vi "GageComplexTriggerAcquire.vi"() -> ()   [LabVIEW 2015]
panel:
  in  "Force":bool
  in  "Trigger Engines":T1(array[cluster])=[{"Slope"=0, "Level"=0, "Source"=0, "External Range"=2000, "External Coupling"=0, "External"=FALSE, "Disable"=FALSE, "External Impedance"=1}] {"External Impedance" items=["50 Ohm", "HiZ"]; "External Coupling" items=["DC", "AC"]; "External Range" min=2000 max=10000 step=8000; "Slope" items=["Rising", "Falling"]; "Level" min=-100 max=100; "Source" min=0 max=64 step=1}
  in  "Channels":T2(array[cluster])=[{"Coupling"=0, "Differential Input"=FALSE, "Direct-to-ADC"=FALSE, "Range"=2000, "Impedance"=50, "DC Offset"=0, "Filter"=0}] {"Impedance" min=50 max=1000000 step=999950; "Coupling" items=["DC", "AC"]}
  in  "Acquisition":T3={"Sample Rate"=100000000.0, "Mode"=0, "Depth"=8192.0, "Segment Size"=8192.0, "Trigger Timeout"=1000000.0, "Trigger Holdoff"=0.0, "Trigger Delay"=0.0, "Clock mode"=enum."Internal"} {"Segment Size" min=256.0 step=128.0; "Trigger Delay" min=0.0 step=128.0; "Trigger Holdoff" min=0.0 step=128.0; "Depth" min=256.0 step=128.0; "Mode" items=["Single", "Dual", "Quad", "Octal"]}
  in  "Continuous":bool
  out "Progress":string
  in  "stop":bool
  out "Waveform Graph":cluster{dbl, dbl, "Data in Volts":dbl[][]}(graph)
  out "System Name":string
  out "Sample Bits":i32
  out "Trigger Count":i32
  out "Channel Count":i32
  out "Board Count":i32
  out "System Count":i32
  in  "Points":u32=4096
  in  "Start":i32
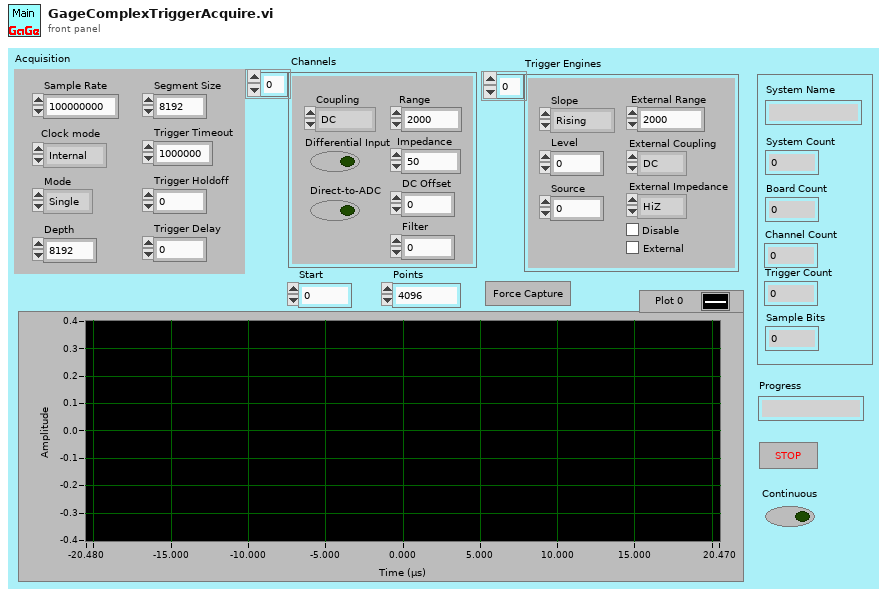
[diagram p1: front panel]
types:
  T1 = cluster{"Slope":u16, "Level":i32, "Source":i32, "External Range":u32, "External Coupling":u16, "External":bool, "Disable":bool, "External Impedance":u16}[]
  T2 = cluster{"Coupling":u16, "Differential Input":bool, "Direct-to-ADC":bool, "Range":u32, "Impedance":u32, "DC Offset":i32, "Filter":i32}[]
  T3 = cluster{"Sample Rate":dbl, "Mode":u16, "Depth":dbl, "Segment Size":dbl, "Trigger Timeout":dbl, "Trigger Holdoff":dbl, "Trigger Delay":dbl, "Clock mode":enum16{"Internal", "External", "Reference"}}
  T4 = cluster{"Handle":u32, "Sample size":u32, "Resolution":i32, "Offset":i32, "Channels":u32, "Boards":u32}
  T5 = cluster{"Slope":u16, "Level":i32, "Source":i32, "External Range":u32, "External Coupling":u16, "External":bool, "Disable":bool, "External Impedance":u16}
  T6 = cluster{"Coupling":u16, "Differential Input":bool, "Direct-to-ADC":bool, "Range":u32, "Impedance":u32, "DC Offset":i32, "Filter":i32}
  T7 = cluster{string, "Level":i32, "Source":i32, "External Range":u32, string, "External":bool, "Disable":bool, string}
  T8 = cluster{string, "Differential Input":bool, "Direct-to-ADC":bool, "Range":u32, "Impedance":u32, "DC Offset":i32, "Coupling":u16}
  T9 = cluster{"Sample Rate":dbl, "Clock mode":enum16{"Internal", "External", "Reference"}, "RingText.Text":string, "Depth":dbl, "Segment Size":dbl, "Trigger Timeout":dbl, "Trigger Holdoff":dbl, "Trigger Delay":dbl}
  T10 = cluster{"Handle":u32, "Sample Size":u32, "Resolution":i32, "Offset":i32, "Channels":u32, "Boards":u32}
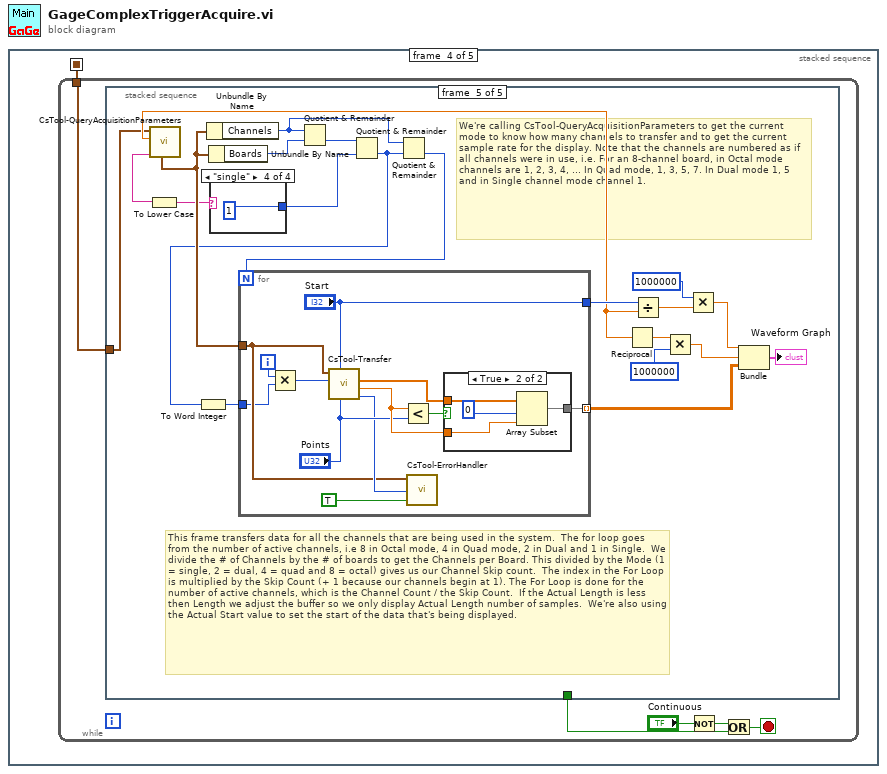
[diagram p0: block diagram]
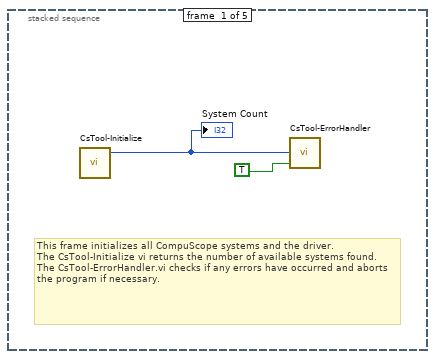
[diagram p2: hidden frame]
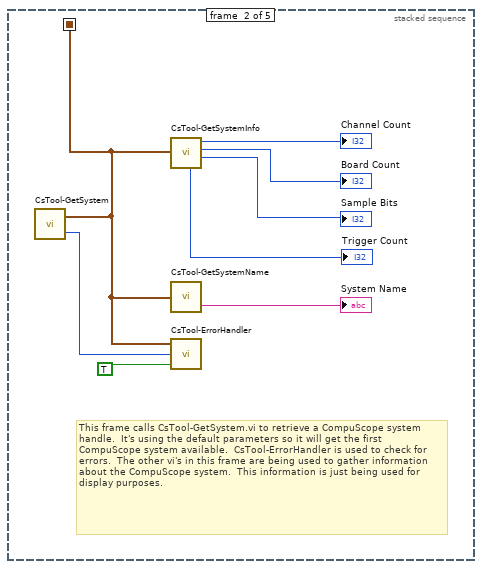
[diagram p3: hidden frame]
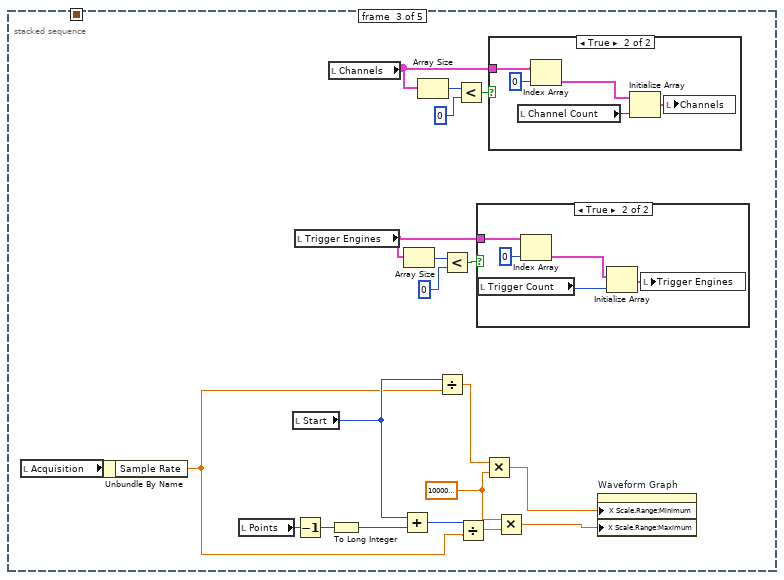
[diagram p4: hidden frame]
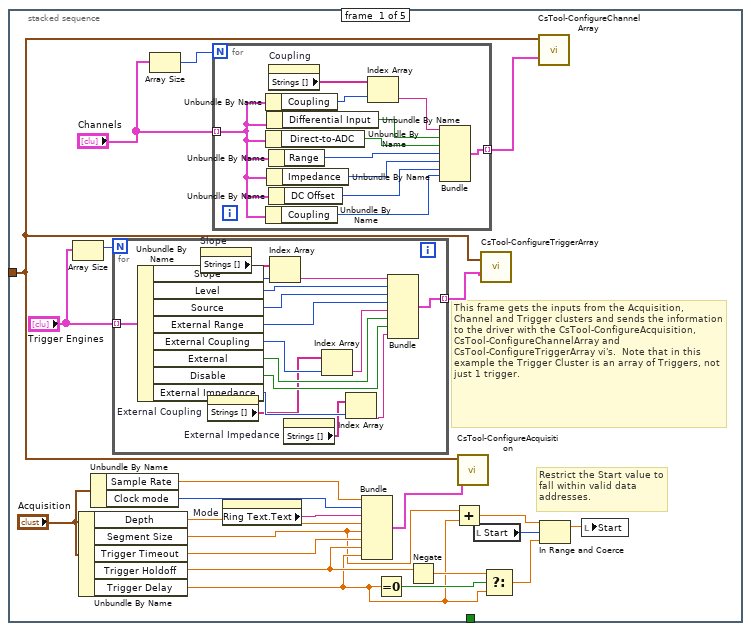
[diagram p7: hidden frame]
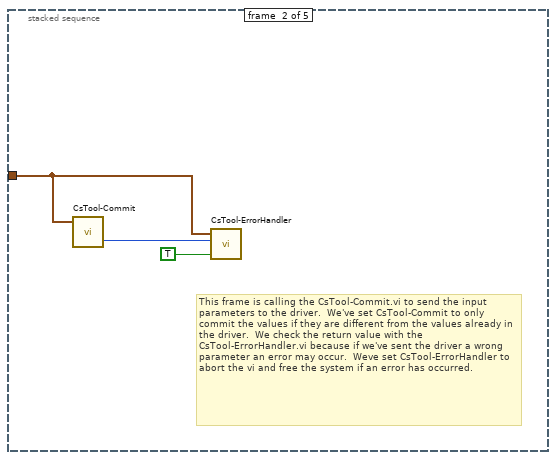
[diagram p8: hidden frame]
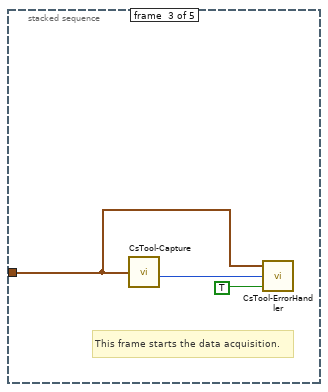
[diagram p9: hidden frame]
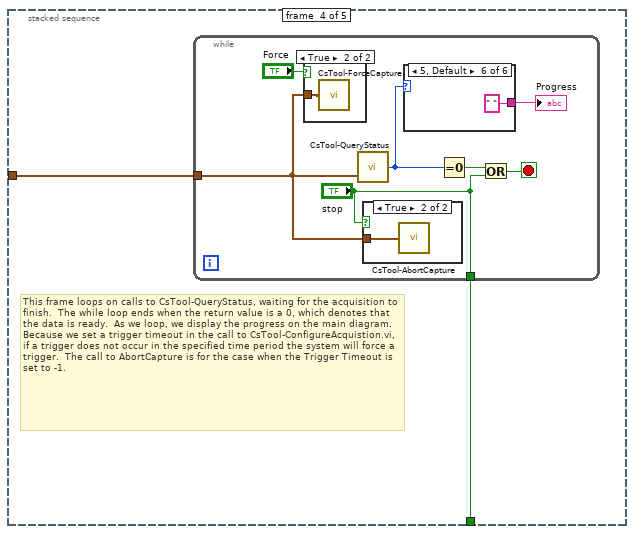
[diagram p10: hidden frame]
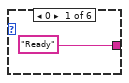
[diagram p13: hidden frame]
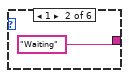
[diagram p14: hidden frame]
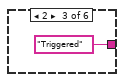
[diagram p15: hidden frame]
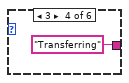
[diagram p16: hidden frame]
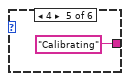
[diagram p17: hidden frame]
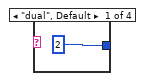
[diagram p18: hidden frame]
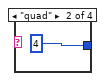
[diagram p19: hidden frame]
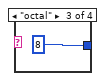
[diagram p20: hidden frame]
diagram:
  n1 = stacked-sequence {
    seq-local: [_ w5 _ _ _] -> [_ _ _ w41 w162]
    frame #0 {
      # "This frame initializes all CompuScope systems and the driver.\nThe CsTool-Initialize vi returns the number of available systems found.  The CsTool-ErrorHandler.vi checks if any errors have occurred and aborts the program if necessary."
      n2 = call <userlib>:"CsTool-Initialize.vi"() -> ("Number Of Systems"=w2:i32)  [unwired: 1 out]
      "System Count" <- w2
      n3 = call <userlib>:"CsTool-ErrorHandler.vi"("StopOnError (true)"=TRUE, "Error Code"=w2) -> ()  [unwired: 1 in, 1 out]
    }
    frame #1 {
      # "This frame calls CsTool-GetSystem.vi to retrieve a CompuScope system handle.  It's using the default parameters so it will get the first CompuScope system available.  CsTool-ErrorHandler is used to check for errors.  The other vi's in this frame are being used to gather information about the CompuScope system.  This information is just being used for display purposes."
      n4 = call <userlib>:"CsTool-GetSystem.vi"() -> ("Error Code"=w7:i32, "Handle Cluster"=w5:T4)  [unwired: 4 in]
      n5 = call <userlib>:"CsTool-GetSystemInfo.vi"("Handle Cluster"=w5) -> ("Number Of Triggers"=→"Trigger Count":u32, "Number Of Channels"=→"Channel Count":u32, "Number Of Boards"=→"Board Count":u32, "Sample Bits"=→"Sample Bits":u32)  [unwired: 3 out]
      n6 = call <userlib>:"CsTool-GetSystemName.vi"("Handle Cluster"=w5) -> ("System Name"=→"System Name":string)  [unwired: 1 out]
      n7 = call <userlib>:"CsTool-ErrorHandler.vi"("StopOnError (true)"=TRUE, "Error Code"=w7, "Handle Cluster"=w5) -> ()  [unwired: 1 out]
    }
    frame #2 {
      w24 = 1000000.0
      n8 = local read "Acquisition"() -> (w22:T3)
      n9 = Unbundle By Name(w22) -> ("Sample Rate"=w21:dbl)
      n10 = local read "Points"() -> (w28:u32)
      n11 = local read "Start"() -> (w27:i32)
      n12 = local read "Trigger Engines"() -> (w13:T1)
      n13 = Decrement(x=w28) -> (x-1=w11:u32)
      n14 = local read "Channels"() -> (w18:T2)
      n15 = To Long Integer(number=w11) -> (32bit integer=w12:i32)
      n16 = Add(x=w27, y=w12) -> (x+y=w29:i32)
      n17 = Array Size(array=w13) -> (size(s)=w15:i32)
      n18 = Array Size(array=w18) -> (size(s)=w19:i32)
      n19 = Divide(x=w27, y=w21) -> (x/y=w30:dbl)
      n20 = Less?(x=w15, y=0) -> (x < y?=w16:bool)
      n21 = Less?(x=w19, y=0) -> (x < y?=w20:bool)
      n22 = Divide(x=w29, y=w21) -> (x/y=w23:dbl)
      n23 = case shown="True" w16 {
        tunnel: w13 -> [_ w33]
        frame False {
        }
        frame True {
          n24 = local read "Trigger Count"() -> (w32:i32)
          n25 = Index Array(array=w33, index=0) -> (element=w34:T5)
          n26 = Initialize Array(w34, w32) -> (w31:T1)
          n27 = local write "Trigger Engines"(w31) -> ()
        }
      }
      n28 = Multiply(x=w30, y=w24) -> (x*y=w26:dbl)
      n29 = case shown="True" w20 {
        tunnel: w18 -> [_ w39]
        frame False {
        }
        frame True {
          n30 = local read "Channel Count"() -> (w38:i32)
          n31 = Index Array(array=w39, index=0) -> (element=w37:T6)
          n32 = Initialize Array(w37, w38) -> (w36:T2)
          n33 = local write "Channels"(w36) -> ()
        }
      }
      n34 = Multiply(x=w24, y=w23) -> (x*y=w25:dbl)
      n35 = property on="Waveform Graph" class="WFGraph (strict)"("X Scale.Range:Minimum"=w26, "X Scale.Range:Maximum"=w25) -> ()  [unwired: 2 in, 2 out]
    }
    frame #3 {
      n36 = while {
        tunnel: w41 -> [w46]
        stop <- w43 stop-if-true
        n37 = stacked-sequence {
          tunnel: w46 -> [w60 w97 w100 w104 w130]
          tunnel: [_ _ _ w103 _] -> w42
          frame #0 {
            # "Restrict the Start value to fall within valid data addresses."
            # "This frame gets the inputs from the Acquisition, Channel and Trigger clusters and sends the information to the driver with the CsTool-ConfigureAcquisition, CsTool-ConfigureChannelArray and CsTool-ConfigureTriggerArray vi's.  Note that in this example the Trigger Cluster is an array of Triggers, not just 1 trigger."
            n38 = Array Size(array="Trigger Engines") -> (size(s)=w62:i32)
            n39 = Unbundle By Name("Acquisition") -> ("Depth"=w68:dbl, "Segment Size"=w47:dbl, "Trigger Timeout"=w57:dbl, "Trigger Holdoff"=w49:dbl, "Trigger Delay"=w48:dbl)
            n40 = Unbundle By Name("Acquisition") -> ("Sample Rate"=w58:dbl, "Clock mode"=w69:enum16{"Internal", "External", "Reference"})
            n41 = for {
              N: w62 -> [_]
              tunnel: "Trigger Engines" -> [w81] mode=indexing
              tunnel: [w82] -> w56 mode=indexing
              n42 = Unbundle By Name(w81) -> ("Slope"=w85:u16, "Level"=w80:i32, "Source"=w79:i32, "External Range"=w78:u32, "External Coupling"=w77:u16, "External"=w76:bool, "Disable"=w75:bool, "External Impedance"=w74:u16)
              n43 = property on="Slope" class="Ring (strict)"() -> ("Strings []"=w72:string[])  [unwired: 2 in, 2 out]
              n44 = property on="External Coupling" class="Ring (strict)"() -> ("Strings []"=w70:string[])  [unwired: 2 in, 2 out]
              n45 = Index Array(array=w72, index=w85) -> (element=w84:string)
              n46 = property on="External Impedance" class="Ring (strict)"() -> ("Strings []"=w71:string[])  [unwired: 2 in, 2 out]
              n47 = Index Array(array=w70, index=w77) -> (element=w83:string)
              n48 = Index Array(array=w71, index=w74) -> (element=w73:string)
              n49 = Bundle(w84, "Level"=w80, "Source"=w79, "External Range"=w78, w83, "External"=w76, "Disable"=w75, w73) -> (w82:T7)  [unwired: 1 in]
            }
            n50 = Array Size(array="Channels") -> (size(s)=w67:i32)
            n51 = for {
              N: w67 -> [_]
              tunnel: "Channels" -> [w87] mode=indexing
              tunnel: [w91] -> w63 mode=indexing
              n52 = Unbundle By Name(w87) -> ("Coupling"=w90:u16)
              n53 = Unbundle By Name(w87) -> ("Direct-to-ADC"=w95:bool)
              n54 = Unbundle By Name(w87) -> ("Coupling"=w86:u16)
              n55 = Unbundle By Name(w87) -> ("Differential Input"=w96:bool)
              n56 = Unbundle By Name(w87) -> ("Impedance"=w93:u32)
              n57 = property on="Coupling" class="Ring (strict)"() -> ("Strings []"=w88:string[])  [unwired: 2 in, 2 out]
              n58 = Unbundle By Name(w87) -> ("Range"=w94:u32)
              n59 = Unbundle By Name(w87) -> ("DC Offset"=w92:i32)
              n60 = Index Array(array=w88, index=w90) -> (element=w89:string)
              n61 = Bundle(w89, "Differential Input"=w96, "Direct-to-ADC"=w95, "Range"=w94, "Impedance"=w93, "DC Offset"=w92, "Coupling"=w86) -> (w91:T8)  [unwired: 1 in]
            }
            n62 = property on="Mode" class="Ring (strict)"() -> ("Ring Text.Text"=w65:string)  [unwired: 2 in, 2 out]
            n63 = Bundle("Sample Rate"=w58, "Clock mode"=w69, "RingText.Text"=w65, "Depth"=w68, "Segment Size"=w47, "Trigger Timeout"=w57, "Trigger Holdoff"=w49, "Trigger Delay"=w48) -> (w64:T9)  [unwired: 1 in]
            n64 = Equal To 0?(x=w48) -> (x = 0?=w50:bool)
            n65 = Negate(x=w49) -> (-x=w51:dbl)
            n66 = Add(x=w47, y=w48) -> (x+y=w53:dbl)
            n67 = call <userlib>:"CsTool-ConfigureAcquisition.vi"("Handle Cluster"=w60, "Acquisition"=w64) -> ()  [unwired: 3 in, 1 out]
            n68 = local read "Start"() -> (w54:i32)
            n69 = call <userlib>:"CsTool-ConfigureTriggerArray.vi"("Triggers"=w56, "Handle Cluster"=w60) -> ()  [unwired: 1 out]
            n70 = Select(t=w51, s=w50, f=w48) -> (s? t:f=w52:dbl)
            n71 = call <userlib>:"CsTool-ConfigureChannelArray.vi"("Channels"=w63, "Handle Cluster"=w60) -> ()  [unwired: 1 out]
            n72 = In Range and Coerce(upper limit=w53, x=w54, lower limit=w52) -> (coerced(x)=w55:dbl)  [unwired: 1 out]
            n73 = local write "Start"(w55) -> ()
          }
          frame #1 {
            # "This frame is calling the CsTool-Commit.vi to send the input parameters to the driver.  We've set CsTool-Commit to only commit the values if they are different from the values already in the driver.  We check the return value with the CsTool-ErrorHandler.vi because if we've sent the driver a wrong parameter an error may occur.  Weve set CsTool-ErrorHandler to abort the vi and free the system if an error has occurred."
            n74 = call <userlib>:"CsTool-Commit.vi"("Handle Cluster"=w97) -> ("Error Code"=w99:i32)  [unwired: 2 in, 1 out]
            n75 = call <userlib>:"CsTool-ErrorHandler.vi"("StopOnError (true)"=TRUE, "Error Code"=w99, "Handle Cluster"=w97) -> ()  [unwired: 1 out]
          }
          frame #2 {
            # "This frame starts the data acquisition."
            n76 = call <userlib>:"CsTool-Capture.vi"("Handle Cluster"=w100) -> ("Error Code"=w102:i32)
            n77 = call <userlib>:"CsTool-ErrorHandler.vi"("StopOnError (true)"=TRUE, "Error Code"=w102, "Handle Cluster"=w100) -> ()  [unwired: 1 out]
          }
          frame #3 {
            # "This frame loops on calls to CsTool-QueryStatus, waiting for the acquisition to finish.  The while loop ends when the return value is a 0, which denotes that the data is ready.  As we loop, we display the progress on the main diagram.  Because we set a trigger timeout in the call to CsTool-ConfigureAcquistion.vi, if a trigger does not occur in the specified time period the system will force a trigger.  The call to AbortCapture is for the case when the Trigger Timeout is set to -1."
            n78 = while {
              tunnel: w104 -> [w106]
              tunnel: ["stop"] -> w103
              stop <- w108 stop-if-true
              n79 = case shown="True" "Force" {
                tunnel: w106 -> [_ w112]
                frame False {
                }
                frame True {
                  n80 = call "CsTool-ForceCapture.vi"("Handle Cluster"=w112) -> ()  [unwired: 1 out]
                }
              }
              n81 = call <userlib>:"CsTool-QueryStatus.vi"("Handle Cluster"=w106) -> ("Status"=w111:i32)
              n82 = case shown="True" "stop" {
                tunnel: w106 -> [_ w113]
                frame False {
                }
                frame True {
                  n83 = call <userlib>:"CsTool-AbortCapture.vi"("Handle Cluster"=w113) -> ()  [unwired: 1 out]
                }
              }
              n84 = case shown="5, Default" w111 {
                tunnel: ["Ready" "Waiting" "Triggered" "Transferring" "Calibrating" " "] -> w110
                frame 0 {
                }
                frame 1 {
                }
                frame 2 {
                }
                frame 3 {
                }
                frame 4 {
                }
                frame 5, Default {
                }
              }
              "Progress" <- w110
              n85 = Equal To 0?(x=w111) -> (x = 0?=w109:bool)
              n86 = Or(x=w109, y="stop") -> (x .or. y?=w108:bool)
            }
          }
          frame #4 {
            # "We're calling CsTool-QueryAcquisitionParameters to get the current mode to know how many channels to transfer and to get the current sample rate for the display. Note that the channels are numbered as if all channels were in use, i.e. For an 8-channel board, in Octal mode channels are 1, 2, 3, 4, ... In Quad mode, 1, 3, 5, 7. In Dual mode 1, 5 and in Single channel mode channel 1."
            # "This frame transfers data for all the channels that are being used in the system.  The for loop goes from the number of active channels, i.e 8 in Octal mode, 4 in Quad mode, 2 in Dual and 1 in Single.  We divide the # of Channels by the # of boards to get the Channels per Board. This divided by the Mode (1 = single, 2 = dual, 4 = quad and 8 = octal) gives us our Channel Skip count.  The index in the For Loop is multiplied by the Skip Count (+ 1 because our channels begin at 1). The For Loop is done for the number of active channels, which is the Channel Count / the Skip Count.  If the Actual Length is less then Length we adjust the buffer so we only display Actual Length number of samples.  We're also using the Actual Start value to set the start of the data that's being displayed."
            n87 = call <userlib>:"CsTool-QueryAcquisitionParameters.vi"("Handle Cluster"=w130) -> ("Output Handle Cluster"=w129:T10, "Mode"=w127:string, "Sample Rate"=w131:dbl)  [unwired: 8 out]
            n88 = To Lower Case(string=w127) -> (all lower case string=w126:string)
            n89 = Unbundle By Name(w129) -> ("Channels"=w122:u32)
            n90 = Unbundle By Name(w129) -> ("Boards"=w125:u32)
            n91 = case shown="\"single\"" w126 {
              tunnel: [2 4 8 1] -> w123
              frame "dual", Default {
              }
              frame "quad" {
              }
              frame "octal" {
              }
              frame "single" {
              }
            }
            n92 = Quotient & Remainder(x=w122, y=w125) -> (floor(x/y)=w124:u32)  [unwired: 1 out]
            n93 = Quotient & Remainder(x=w124, y=w123) -> (floor(x/y)=w121:u32)  [unwired: 1 out]
            n94 = To Word Integer(number=w121) -> (16bit integer=w128:i16)
            n95 = Quotient & Remainder(x=w122, y=w121) -> (floor(x/y)=w120:u32)  [unwired: 1 out]
            n96 = for {
              N: w120 -> [_]
              tunnel: ["Start"] -> w135
              tunnel: [w152] -> w134 mode=indexing
              tunnel: w129 -> [w149]
              tunnel: w128 -> [w147]
              i -> [w148]
              n97 = Multiply(x=w148, y=w147) -> (x*y=w146:i32)
              n98 = call <userlib>:"CsTool-Transfer.vi"("Length (4096)"="Points", "Start (0)"="Start", "Channel (0)"=w146, "Handle Cluster"=w149) -> ("Error Code"=w151:i32, "Actual Length"=w155:dbl, "Data in Volts"=w154:dbl[])  [unwired: 2 in, 1 out]
              n99 = Less?(x=w155, y="Points") -> (x < y?=w156:bool)
              n100 = call <userlib>:"CsTool-ErrorHandler.vi"("StopOnError (true)"=TRUE, "Error Code"=w151, "Handle Cluster"=w149) -> ()  [unwired: 1 out]
              n101 = case shown="True" w156 {
                tunnel: w154 -> [w157 w161]
                tunnel: w155 -> [_ w159]
                tunnel: [w157 w158] -> w152
                frame False {
                }
                frame True {
                  n102 = Array Subset(array=w161, index=0, length=w159) -> (w158:dbl[])
                }
              }
            }
            n103 = Reciprocal(x=w131) -> (1/x=w136:dbl)
            n104 = Divide(x=w135, y=w131) -> (x/y=w139:dbl)
            n105 = Multiply(x=w136, y=1000000) -> (x*y=w138:dbl)
            n106 = Multiply(x=1000000, y=w139) -> (x*y=w140:dbl)
            n107 = Bundle(w140, w138, "Data in Volts"=w134) -> (→"Waveform Graph":cluster{dbl, dbl, "Data in Volts":dbl[][]})  [unwired: 1 in]
          }
        }
        n108 = Not(x="Continuous") -> (.not. x?=w45:bool)
        n109 = Or(x=w45, y=w42) -> (x .or. y?=w43:bool)
      }
    }
    frame #4 {
      # "This frame frees the handle associated with the CompuScope system we've been using.  This allows the system to be used by another application."
      n110 = call "CsTool-FreeSystem.vi"("Handle Cluster"=w162) -> ()  [unwired: 1 out]
    }
  }
